vi "Voice Select.vi"(11 "Voice name":string) -> (3 "Voice":i32)   [LabVIEW 2017]
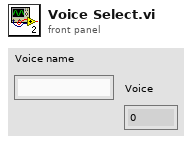
[diagram p1: front panel]
types:
  T1 = cluster{i32, "Description":string, "Name":string, "TwoLetterISOLanguageName":string}[]
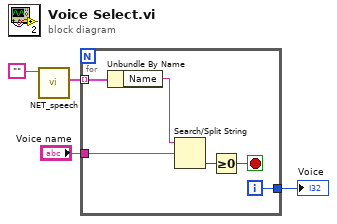
[diagram p0: block diagram]
diagram:
  n1 = call "NET_speech.vi"("textToSpeak"="") -> ("Голоса"=w2:T1)  [unwired: 2 in, 8 out]
  n2 = for {
    tunnel: w2 -> [w10] mode=indexing
    tunnel: "Voice name" -> [w8]
    tunnel: [w5] -> w3
    i -> [w5]
    stop <- w6 stop-if-true
    n3 = Unbundle By Name(w10) -> ("Name"=w9:string)
    n4 = Search/Split String(string=w9, search string/char (-)=w8) -> (offset of match=w7:i32)  [unwired: 1 in, 2 out]
    n5 = Greater Or Equal To 0?(x=w7) -> (x >= 0?=w6:bool)
  }
  "Voice" <- w3
